vi "GetType.vi"(8 "Error In":errorcluster, 11 "Actor Framework:Message in":refnum<class>) -> (0 "Error Out":errorcluster, 2 "Data Sample":variant, 3 "Actor Framework:Message out":refnum<class>)   [LabVIEW 2016]
doc: "(<B>Filename</B>: Actor Framework.lvlib:Message.lvclass:GetType.vi)\n\nReturns a (default) sample of the attribute data needed to create a PV of a this type."
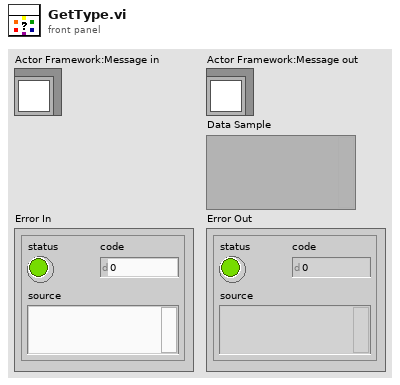
[diagram p1: front panel]
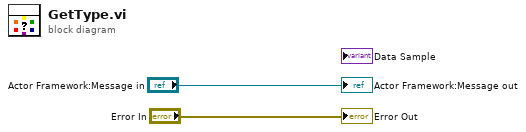
[diagram p0: block diagram]
diagram:
  "Error Out" <- "Error In"
  "Actor Framework:Message out" <- "Actor Framework:Message in"
